vi "Send to Sequencer Core.vi"(7 "In Front?(F)":bool, 8 "error in (no error)":errorcluster, 9 "Message Priority":T1=enum."Normal", 10 "Message Array":refnum<class "Message.lvclass">[](array[class]), 11 "Sequencer in":refnum<class "Sequencer.lvclass">) -> (0 "error out":errorcluster, 3 "Sequencer out":refnum<class "Sequencer.lvclass">)   [LabVIEW 2020, in "Sequencer.lvlib" / "Sequencer.lvclass"]
uses:
  Sequencer.lvclass
  PPL/HDH.Actor Framework.Core.Actor.lvlibp/1abvi3w/vi.lib/ActorFramework/Message Enqueuer/Message Priority.ctl
  PPL/HDH.Actor Framework.Core.Actor.lvlibp/1abvi3w/vi.lib/ActorFramework/Message/Message.lvclass
  Sequencer.lvclass/Sequencer.ctl
  Sequencer Core/Sequencer Core.lvclass/Sequencer Core.ctl
  Sequencer Core/Sequencer Core.lvclass
  PPL/HDH.Actor Framework.Core.Actor.lvlibp/1abvi3w/vi.lib/ActorFramework/Message Enqueuer/Message Enqueuer.lvclass
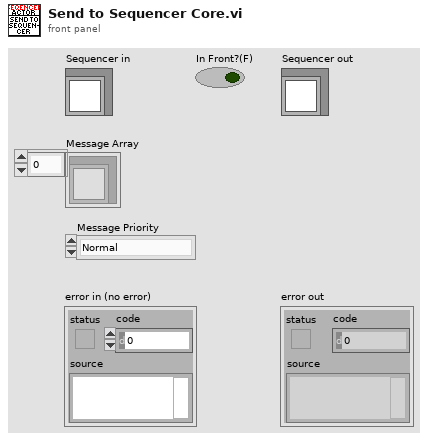
[diagram p1: front panel]
types:
  T1 = typedef "HDH.Actor Framework.Core.Actor.lvlibp/Message Enqueuer.lvclass/Message Priority.ctl" = enum16{"Low", "Normal", "High"}
  T2 = typedef "Semaphore RefNum" = refnum<k1>
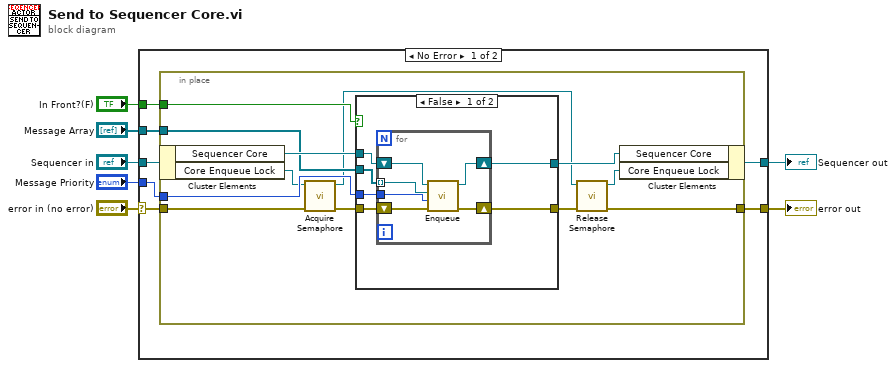
[diagram p0: block diagram]
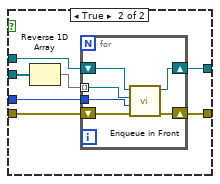
[diagram p2: hidden frame]
diagram:
  n1 = case shown="No Error" "error in (no error)" {
    selector: "error in (no error)" -> [w10 w53]
    tunnel: [w9 w53] -> w6
    tunnel: [w11 w52] -> w4
    tunnel: "Sequencer in" -> [w12 w52]
    tunnel: "Message Priority" -> [w14 _]
    tunnel: "Message Array" -> [w13 _]
    tunnel: "In Front?(F)" -> [w8 _]
    frame No Error {
      n2 = in-place {
        in-place-border: w14 -> [w25]
        in-place-border: w13 -> [w24]
        in-place-border: w10 -> [w20]
        in-place-border: [w15] -> w9
        in-place-border: w8 -> [w22]
        n3 = in-place-cluster #1(w12) -> ("Sequencer Core"=w26:refnum<class "Sequencer Core.lvclass">, "Core Enqueue Lock"=w21:T2)
        n4 = call <vilib>:"Acquire Semaphore.vi"("error in (no error)"=w20, "semaphore"=w21) -> ("error out"=w19:errorcluster, "semaphore out"=w18:T2)  [unwired: 3 in, 1 out]
        n5 = case shown="False" w22 {
          tunnel: w26 -> [w32 w45]
          tunnel: w25 -> [w31 w42]
          tunnel: w24 -> [w30 w43]
          tunnel: [w29 w44] -> w23
          tunnel: w19 -> [w28 w41]
          tunnel: [w27 w40] -> w16
          frame False {
            n6 = for {
              tunnel: w31 -> [w37]
              tunnel: w30 -> [w36] mode=indexing
              shift-right: [w35] -> w29
              shift-left: w32 -> [w38]
              shift-right: [w33] -> w27
              shift-left: w28 -> [w34]
              n7 = call "Enqueue.vi"("error in (no error)"=w34, "Message Priority"=w37, "Message"=w36, "Sequencer Core in"=w38) -> ("error out"=w33:errorcluster, "Sequencer Core out"=w35:refnum<class "Sequencer Core.lvclass">)  [unwired: 6 in]
            }
          }
          frame True {
            n8 = Reverse 1D Array(array=w43) -> (reversed array=w39:refnum<class "Message.lvclass">[])
            n9 = for {
              tunnel: w39 -> [w49] mode=indexing
              tunnel: w42 -> [w48]
              shift-right: [w50] -> w44
              shift-left: w45 -> [w51]
              shift-right: [w46] -> w40
              shift-left: w41 -> [w47]
              n10 = call "Enqueue in Front.vi"("error in (no error)"=w47, "Message Priority"=w48, "Message"=w49, "Sequencer Core in"=w51) -> ("error out"=w46:errorcluster, "Sequencer Core out"=w50:refnum<class "Sequencer Core.lvclass">)  [unwired: 6 in]
            }
          }
        }
        n11 = call <vilib>:"Release Semaphore.vi"("error in (no error)"=w16, "semaphore"=w18) -> ("error out"=w15:errorcluster, "semaphore out"=w17:T2)  [unwired: 4 in]
        n12 = in-place-cluster #1("Sequencer Core"=w23, "Core Enqueue Lock"=w17) -> (w11:refnum<class "Sequencer.lvclass">)
      }
    }
    frame Error {
    }
  }
  "error out" <- w6
  "Sequencer out" <- w4
